vi "Camera.v8.vi"() -> ()   [LabVIEW 2015]
uses:
  Camera Properties.ctl
  Microscope Settings.ctl
  CameraState.ctl
  ModeEnum.ctl
  Stack_State.ctl
  Stack Track.ctl
  CameraControlTypeDef.ctl
  <vilib>/DAQmx/write.llb/DAQmx Write (Digital 1D Wfm NChan NSamp).vi
  <vilib>/DAQmx/write.llb/DAQmx Write (Analog 1D Wfm NChan NSamp).vi
  <vilib>/DAQmx/create/channels.llb/DAQmx Create Channel (DO-Digital Output).vi
  <vilib>/DAQmx/create/channels.llb/DAQmx Create Channel (AO-Voltage-Basic).vi
  <vilib>/Waveform/WDTOps.llb/WDT Number of Waveform Samples DBL.vi
  <vilib>/DAQmx/configure/timing.llb/DAQmx Timing (Sample Clock).vi
  <vilib>/Waveform/DWDTOps.llb/DWDT Uncompress Digital.vi
  <vilib>/DAQmx/miscellaneous.llb/DAQmx Fill In Error Info.vi
  <vilib>/vision/NI_Vision_Development_Module.lvlib
panel:
  in  "Tab Control":enum32{"Camera Settings", "Recording"}(tab)
  in  "?":bool
  in  "Microscope Settings":T1={"Mode"=enum."XY", "Colour 2"={"Laser"=enum."445", "Filter"=0}, "Slit"={"Scanning Mode"=12.0, "Slit Width /%"=5.0}, "Piezo Position /um"=0.0, "Z Axis Stepping"={"Start"=0.0, "Step"=1.0, "End"=100.0}, "Exposure/ms"=40.0, "ROI"={"Height"=2048.0, "Width"=2048.0, "x"=0.0, "y"=0.0}, "Samples per millisecond"=100.0, "Relax/ms"=10.0, "Readout Direction"=2.0, "Trigger Source"=2.0, "Camera Delay"=11.0} {"Colour 2"."Filter" items=["Empty"=1, ""=2, ""=3, "561"=4, ""=5, "488"=6]; "Z Axis Stepping"."End" min=0.0 max=10.0 step=0.05; "Z Axis Stepping"."Step" min=0.0 max=10.0 step=0.05; "Z Axis Stepping"."Start" min=0.0 max=10.0 step=0.05; "ROI"."y" min=0.0 max=10.0 step=0.05; "ROI"."x" min=0.0 max=10.0 step=0.05; "ROI"."Width" min=0.0 max=10.0 step=0.05; "ROI"."Height" min=0.0 max=10.0 step=0.05; "Camera Delay" min=0.0 max=10.0 step=0.05; "Trigger Source" items=["Internal"=1.0, "External"=2.0]; "Readout Direction" items=["Internal"=1.0, "External"=2.0]; "Slit"."Scanning Mode" items=["Full Frame"=1.0, "Slit Scanning"=12.0]; "Piezo Position /um" min=0.0 max=10.0 step=0.05; "Relax/ms" min=0.0 max=10.0 step=0.05}
  in  "Scan":bool
  in  "Scan Continuously":bool
  out "error IO":errorcluster
  in  "Advanced DCAM Controls":i32(listbox) caption="Multicolumn Listbox"
  in  "Properties":T2=4211904 items=["SENSOR MODE"=4212128, "CCD MODE"=4212384, "READOUT MODE"=4211872, "ACTIVE VIEW INDEX"=4343136, "BITS PER CHANNEL"=4342976, "IMAGE PIXEL TYPE"=4343296, "BINNING"=4215968, "EXPOSURE TIME"=2049184, "CONTRAST GAIN"=3163312, "CONTRAST OFFSET"=3163328, "LIGHT MODE"=2114720, "SENSITIVITY"=2114992, "PHOTON IMAGING MODE"=2115200, "HIGH DYNAMIC RANGE MODE"=3163360, "WHITE BALANCE"=3163568, "TEMPERATURE"=2115232, "TEMPERATURE TARGET"=2115264, "SENSOR COOLER FAN"=2115296, "LINEBUNDLE HEIGHT"=4212192, "MECHANICAL SHUTTER"=2115488, "BACK FOCUS POSITION"=8422304, "TRIGGER CONNECTOR"=1066432, "TRIGGER SOURCE"=1066144, "OUTPUT TRIGGER SOURCE"=1852576, "TRIGGER GLOBAL EXPOSURE"=2049680, "FIRST TRIGGER BEHAVIOR"=2049696, "CHANNEL SYNC"=1852352, "READOUT DIRECTION"=4211904, "PRE HSYNC COUNT"=1852704, "INTERNAL LINE SPEED"=4191408, "INTERNAL LINE INVERVAL"=4191424]
  in  "Array":T1[](array[typedef]) {"Colour 2"."Filter" items=["Empty"=1, ""=2, ""=3, "561"=4, ""=5, "488"=6]; "Z Axis Stepping"."End" min=0.0 max=10.0 step=0.05; "Z Axis Stepping"."Step" min=0.0 max=10.0 step=0.05; "Z Axis Stepping"."Start" min=0.0 max=10.0 step=0.05; "ROI"."y" min=0.0 max=10.0 step=0.05; "ROI"."x" min=0.0 max=10.0 step=0.05; "ROI"."Width" min=0.0 max=10.0 step=0.05; "ROI"."Height" min=0.0 max=10.0 step=0.05; "Camera Delay" min=0.0 max=10.0 step=0.05; "Trigger Source" items=["Internal"=1.0, "External"=2.0]; "Readout Direction" items=["Internal"=1.0, "External"=2.0]; "Slit"."Scanning Mode" items=["Full Frame"=1.0, "Slit Scanning"=12.0]; "Piezo Position /um" min=0.0 max=10.0 step=0.05; "Relax/ms" min=0.0 max=10.0 step=0.05}
  out "Image":T3(plugin-control)
  out "Histogram":T4(graph)
  in  "stop":bool
  in  "Signals Debugger":bool
  in  "Calibration":bool
  in  "MultiD Scan":bool
  in  "Stage Controller":bool
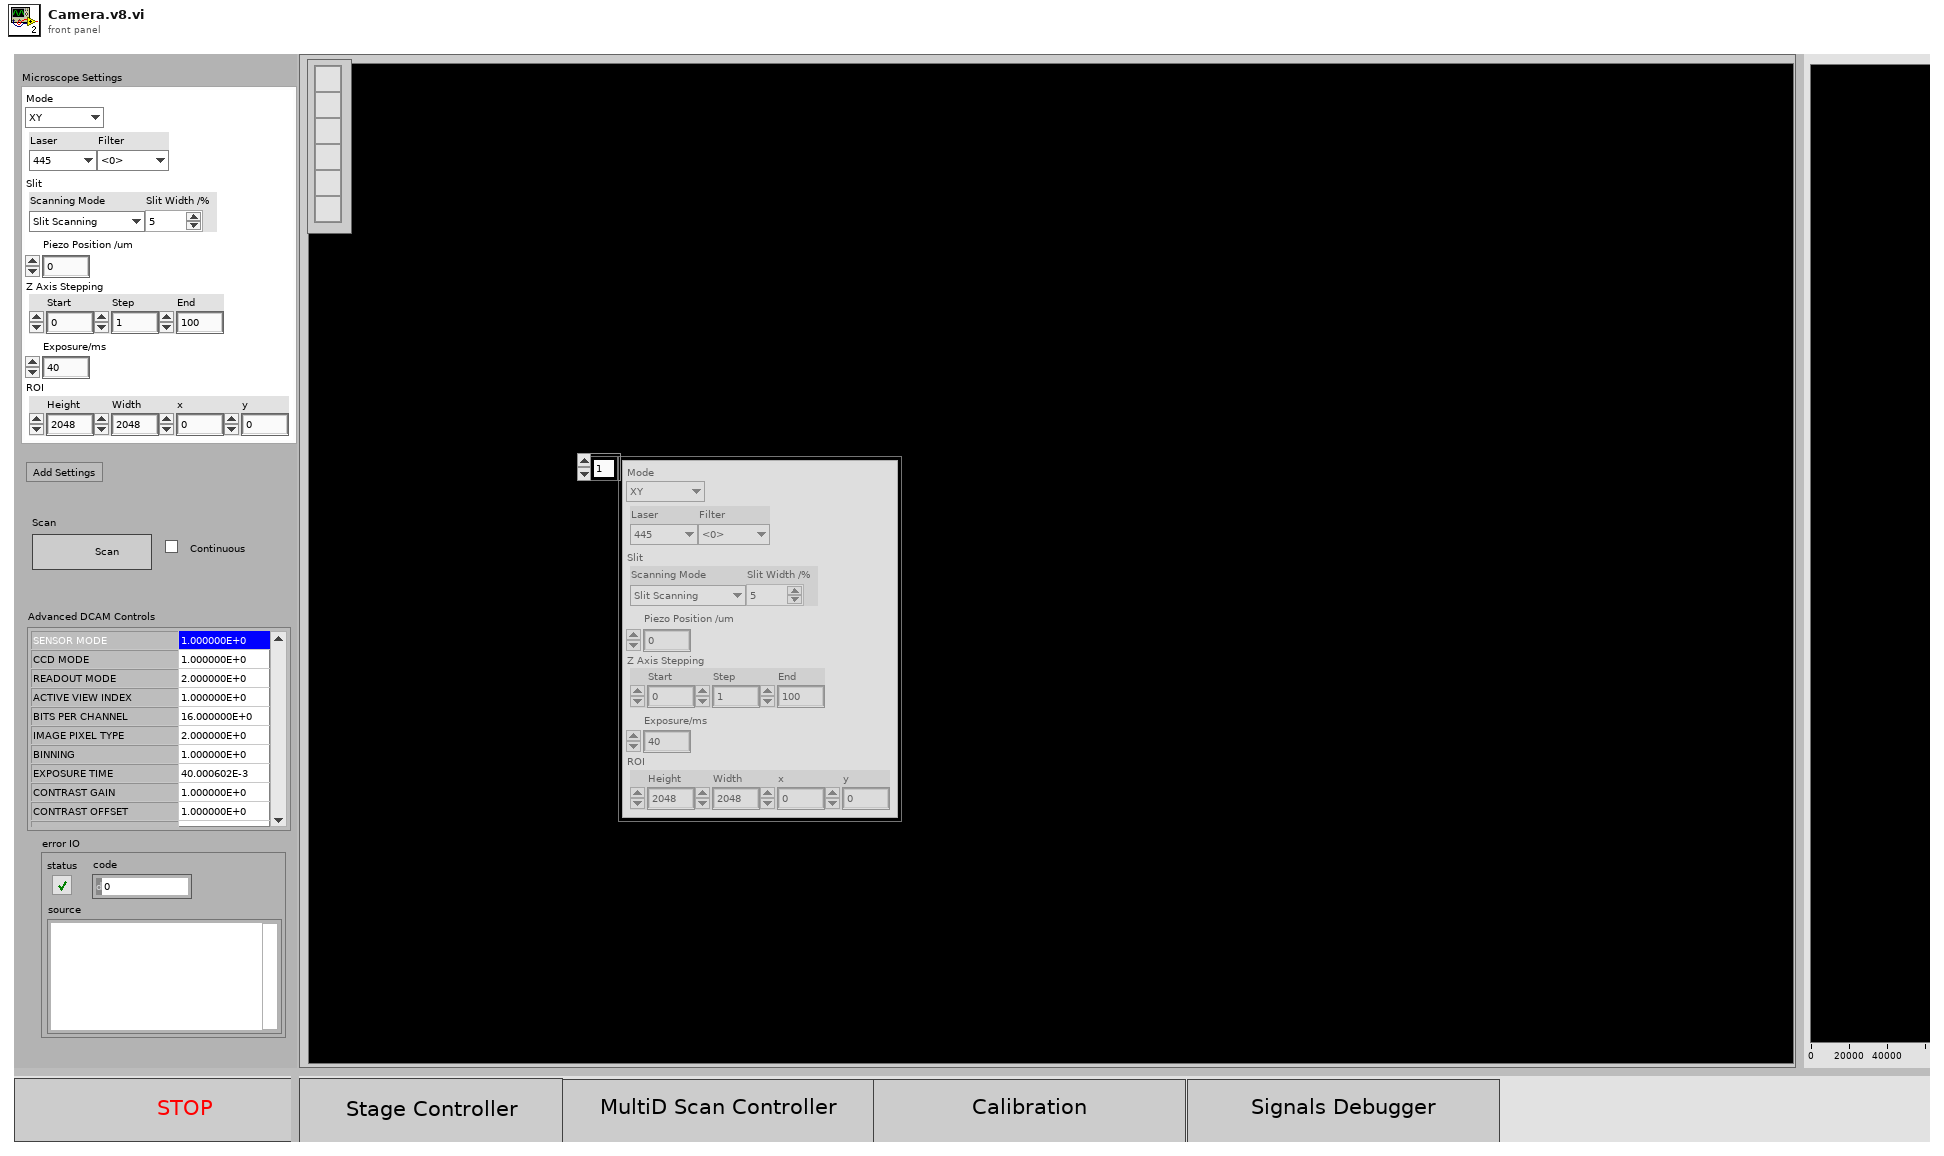
[diagram p1: front panel]
types:
  T1 = typedef "Microscope Settings.ctl" = cluster{"Mode":enum16{"X", "XY", "XYZ", "XYZT", "XYZC"}, "Colour 2":cluster{"Laser":enum16{"445", "488", "561", "647"}, "Filter":u16}, "Slit":cluster{"Scanning Mode":dbl, "Slit Width /%":dbl}, "Piezo Position /um":dbl, "Z Axis Stepping":cluster{"Start":dbl, "Step":dbl, "End":dbl}, "Exposure/ms":dbl, "ROI":cluster{"Height":dbl, "Width":dbl, "x":dbl, "y":dbl}, "Samples per millisecond":dbl, "Relax/ms":dbl, "Readout Direction":dbl, "Trigger Source":dbl, "Camera Delay":dbl}
  T2 = typedef "Camera Properties.ctl" = u32
  T3 = typedef "IMAQ Image.ctl" = refnum<image>
  T4 = cluster{"Starting Value":sgl, "Incremental Value":sgl, "Histogram":u32[]}
  T5 = cluster{"height":u32, "width":u32, "datatype":u32}
  T6 = typedef "CameraState.ctl" = enum16{"init", "active", "deinit"}
  T7 = typedef "ModeEnum.ctl" = enum16{"Idle", "generateWaves", "runWaves", "stop"}
  T8 = typedef "CameraControlTypeDef.ctl" = enum16{"Idle", "IntervalLineInt", "Ram Record", "HardDisk Record", "Disengage Update", "Update", "ROI", "Binning", "Scan Mode", "Trigger Mode", "Readout Mode", "Readout Direction", "Preview", "ROIWindow", "Trigger Source"}
  T9 = cluster{"Mode":u32, "Polarity":u32, "Times":u32, "Delay":dbl}
  T10 = typedef "Stack_State.ctl" = cluster{"State":T11, "Stack Number":i32, "Image":u16[][], "Stacks":i32}
  T11 = typedef "Stack Track.ctl" = enum16{"Idle", "Display", "Start Sequence", "Read Disk", "STOP", "Collecting", "End"}
  T12 = enum32{"Invalid", "Standard", "Closed", "Hidden", "Minimized", "Maximized"}
  T13 = typedef "Image Type" = u32
  T14 = cluster{"State":T11, "Timeout":i32, "Data 16":u16[][], "Timeout":i32}
  T15 = cluster{waveform(dbl)[], "Digital Waveform":digitalwaveform, "Digital Waveform":digitalwaveform}
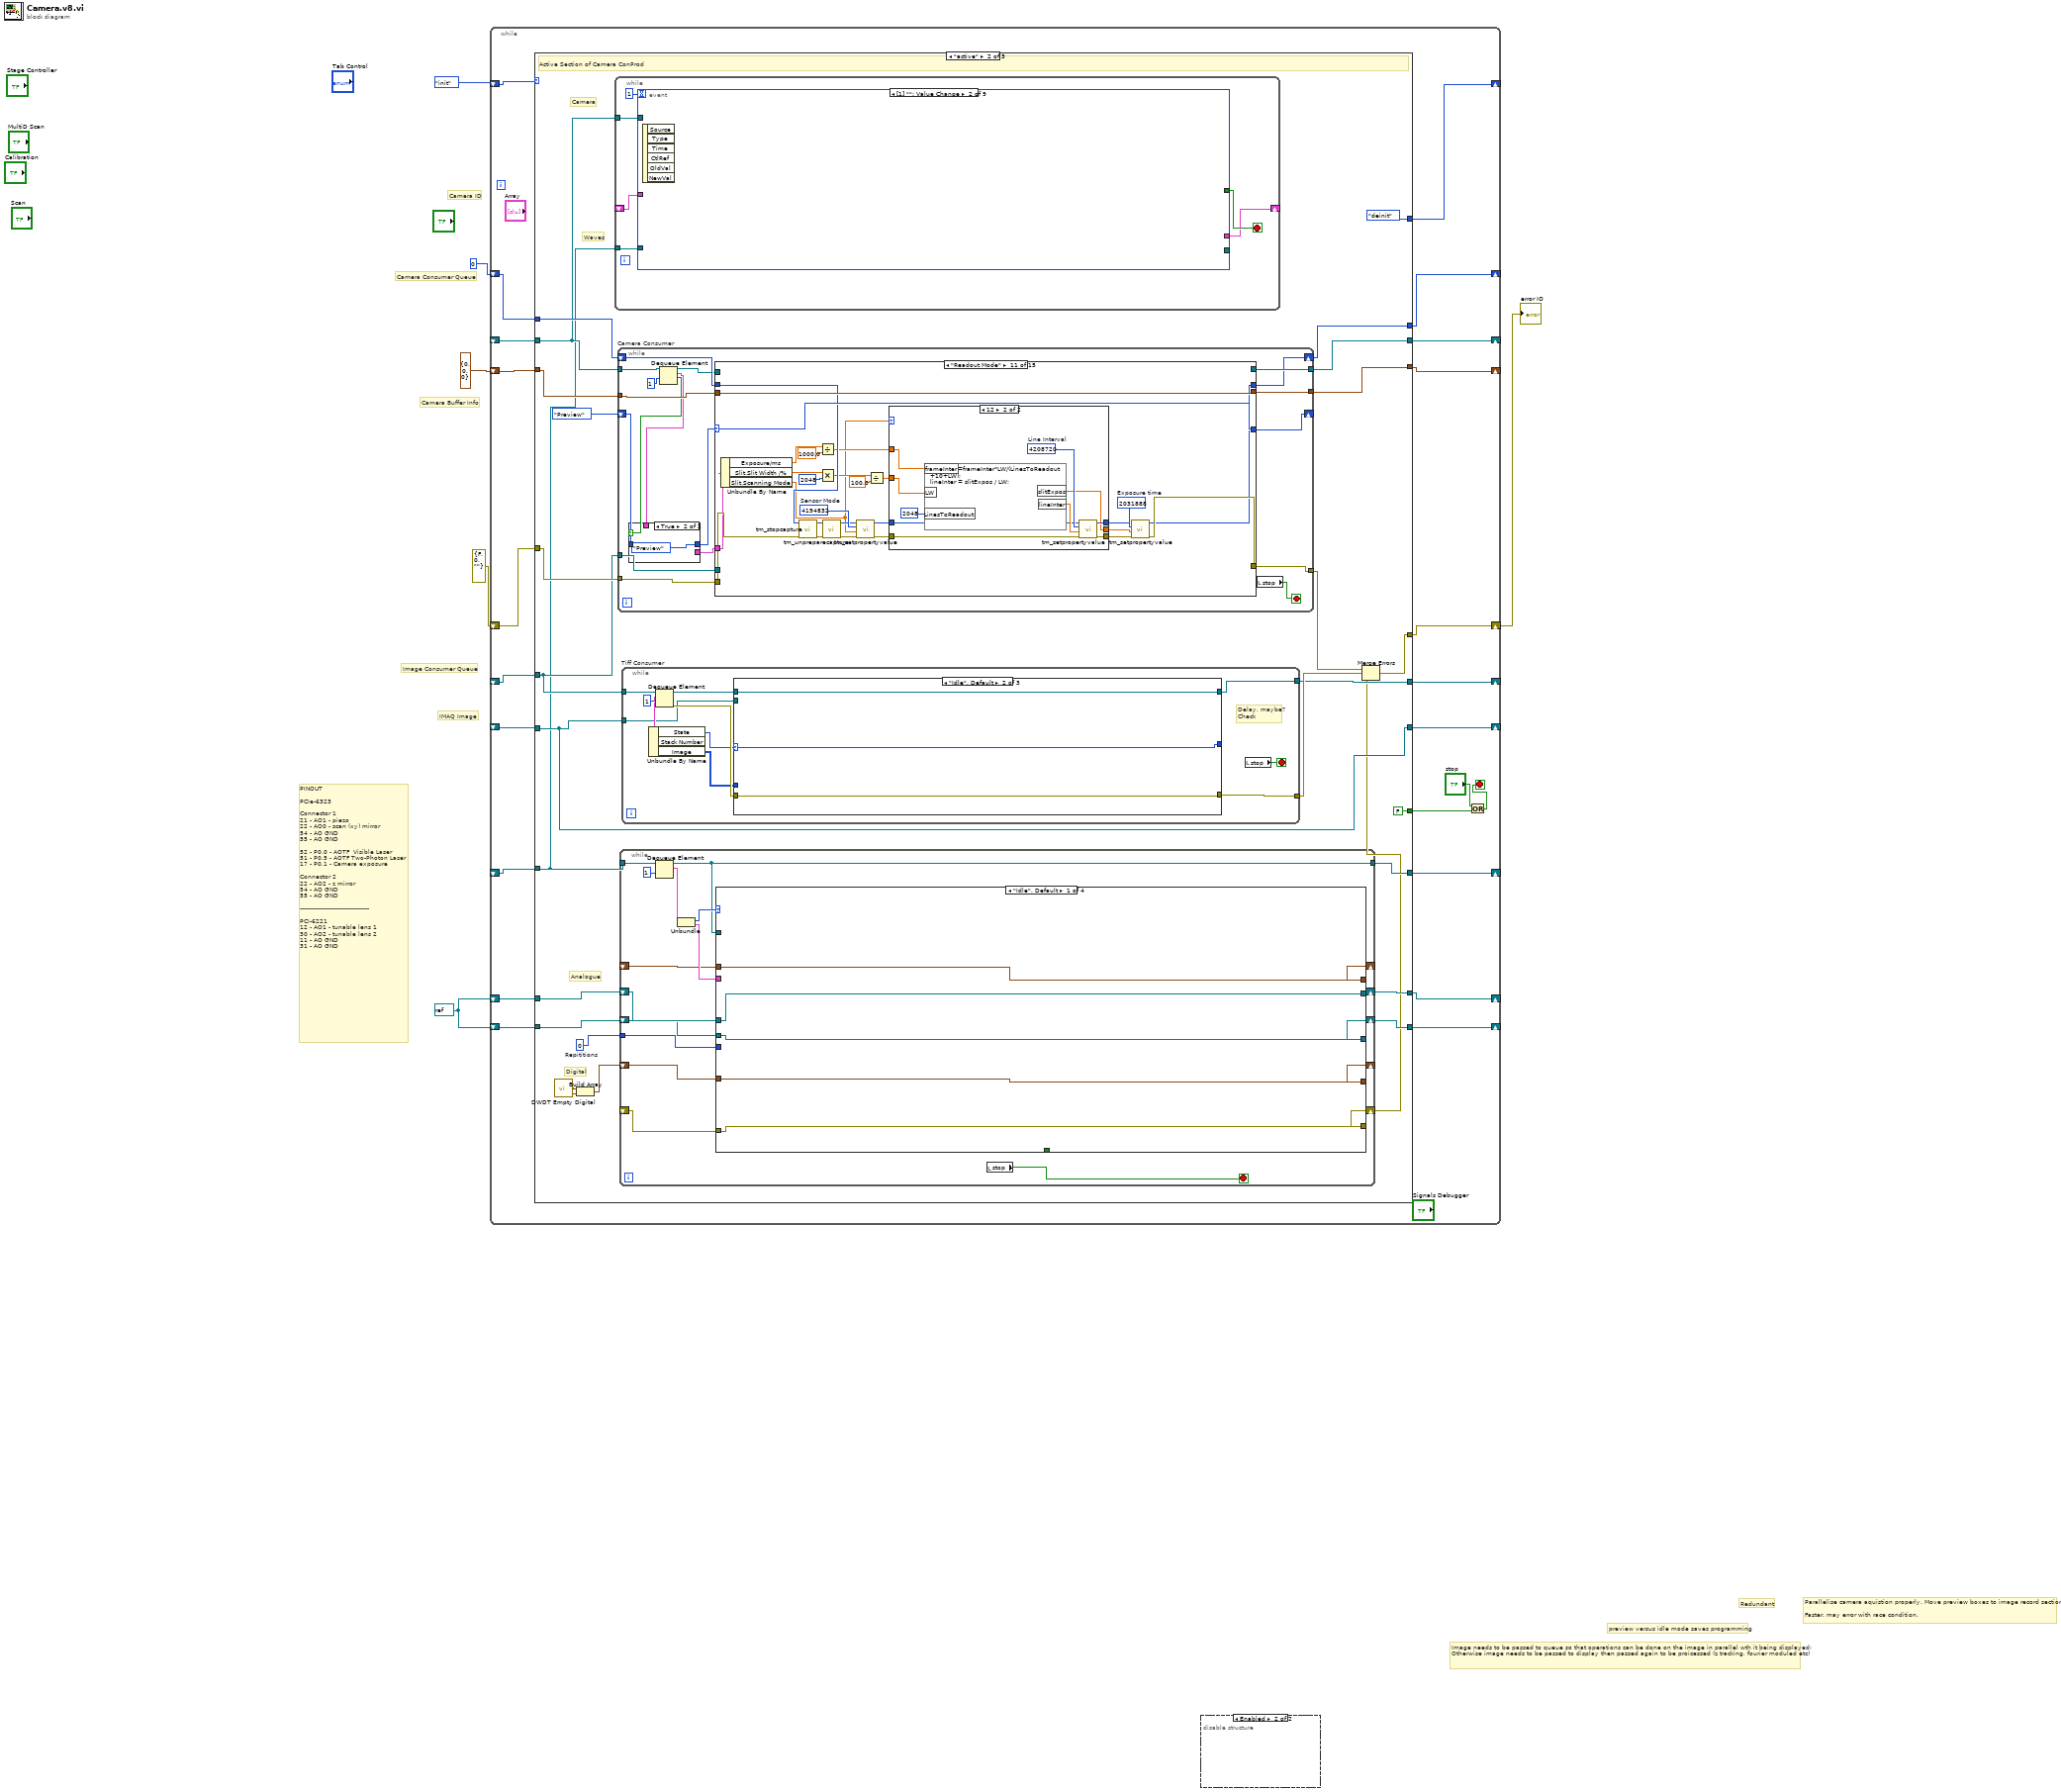
[diagram p0: block diagram]
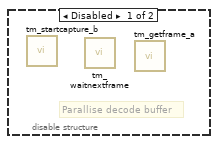
[diagram p2: hidden frame]
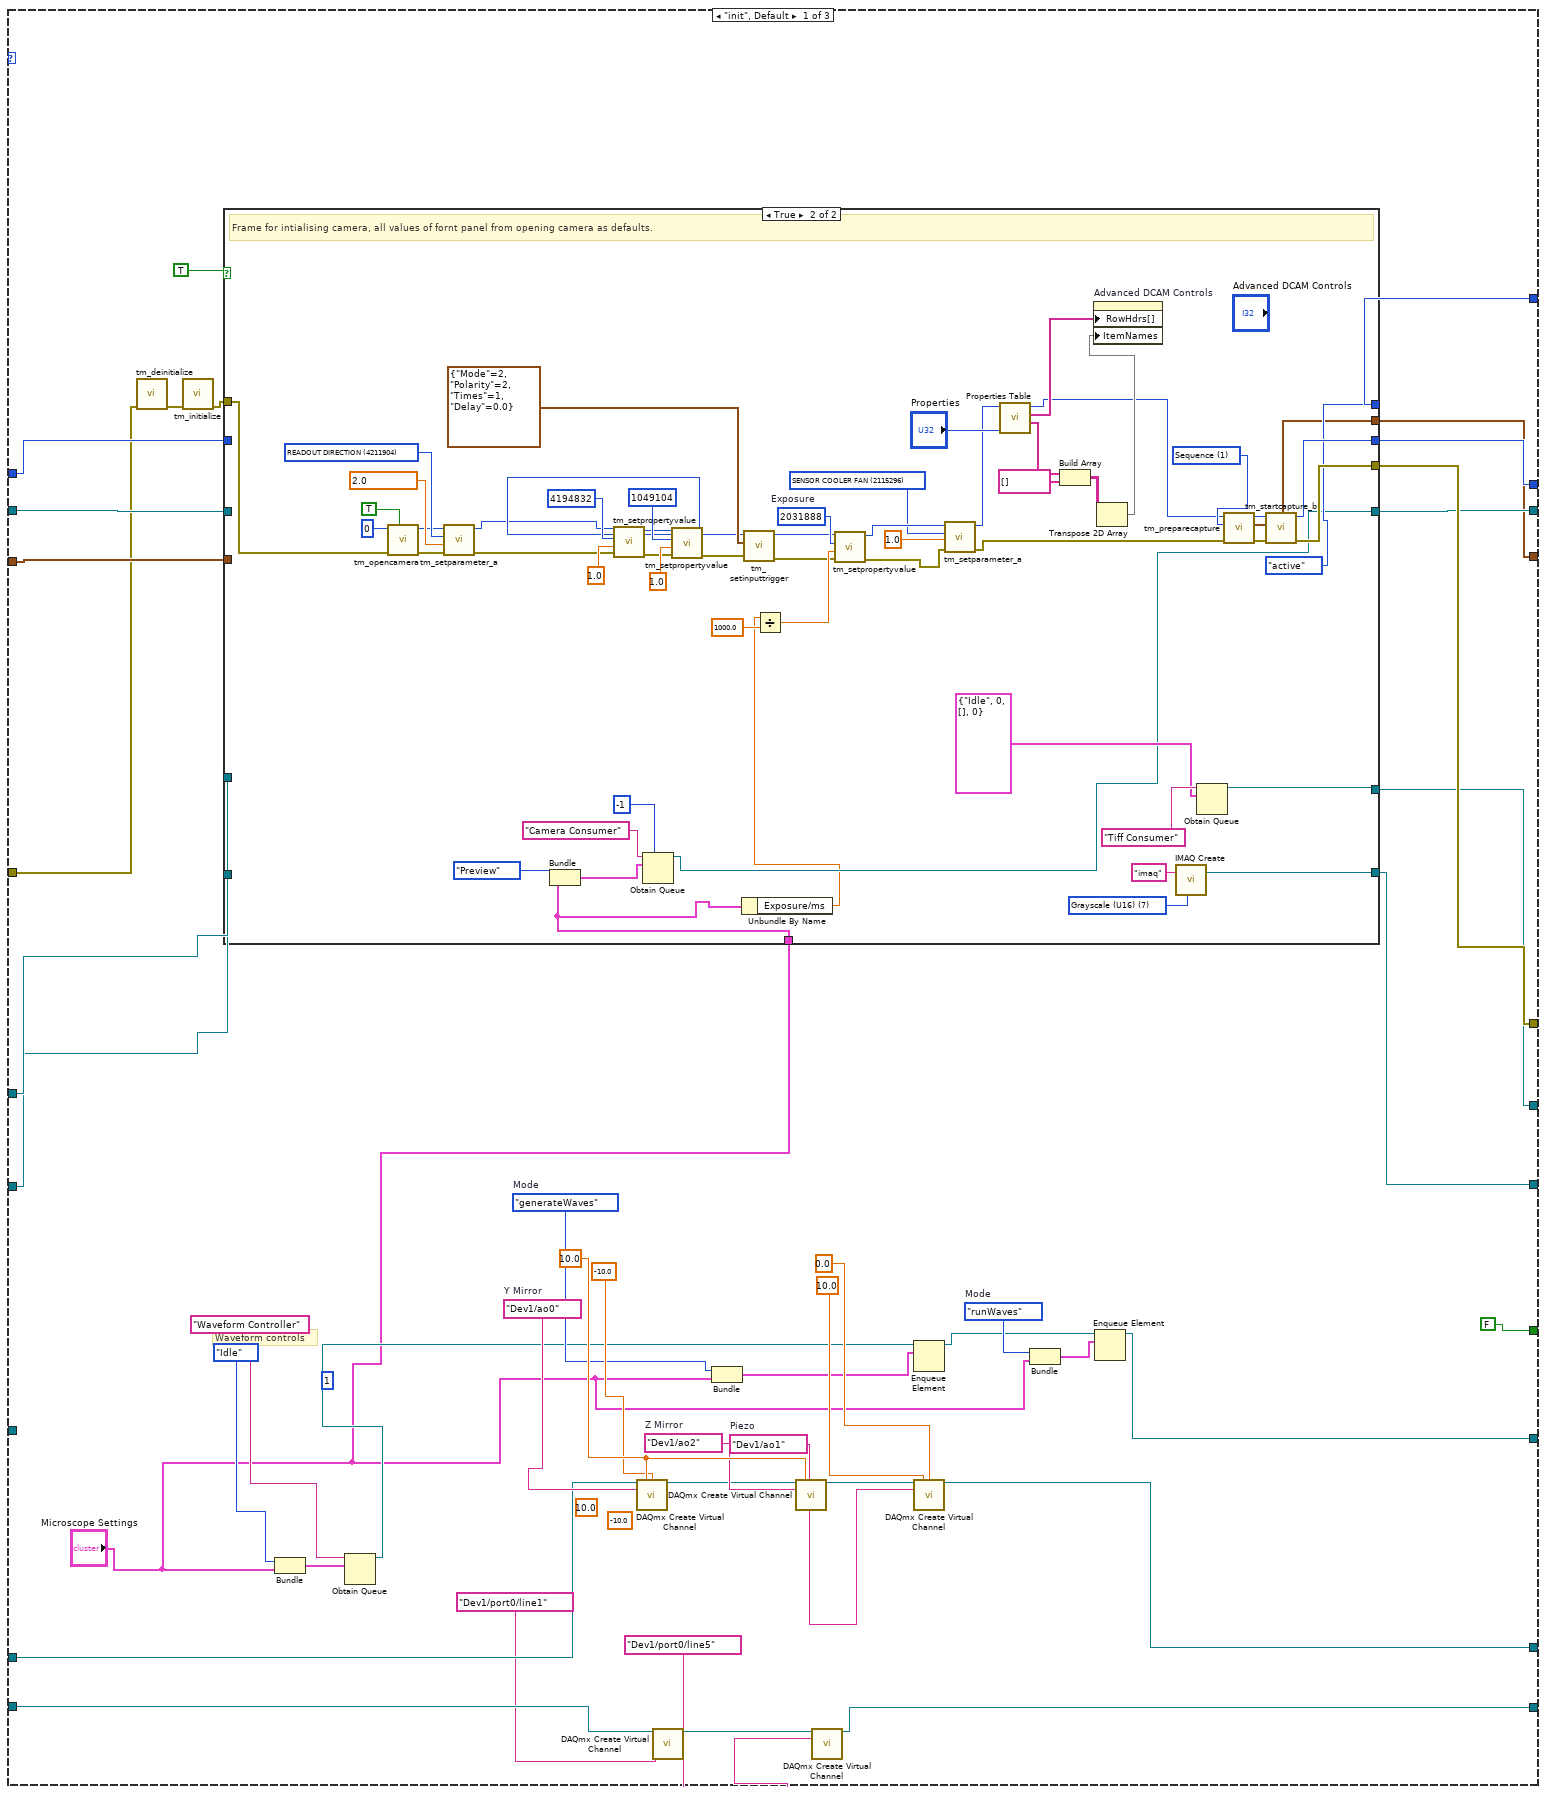
[diagram p3: hidden frame]
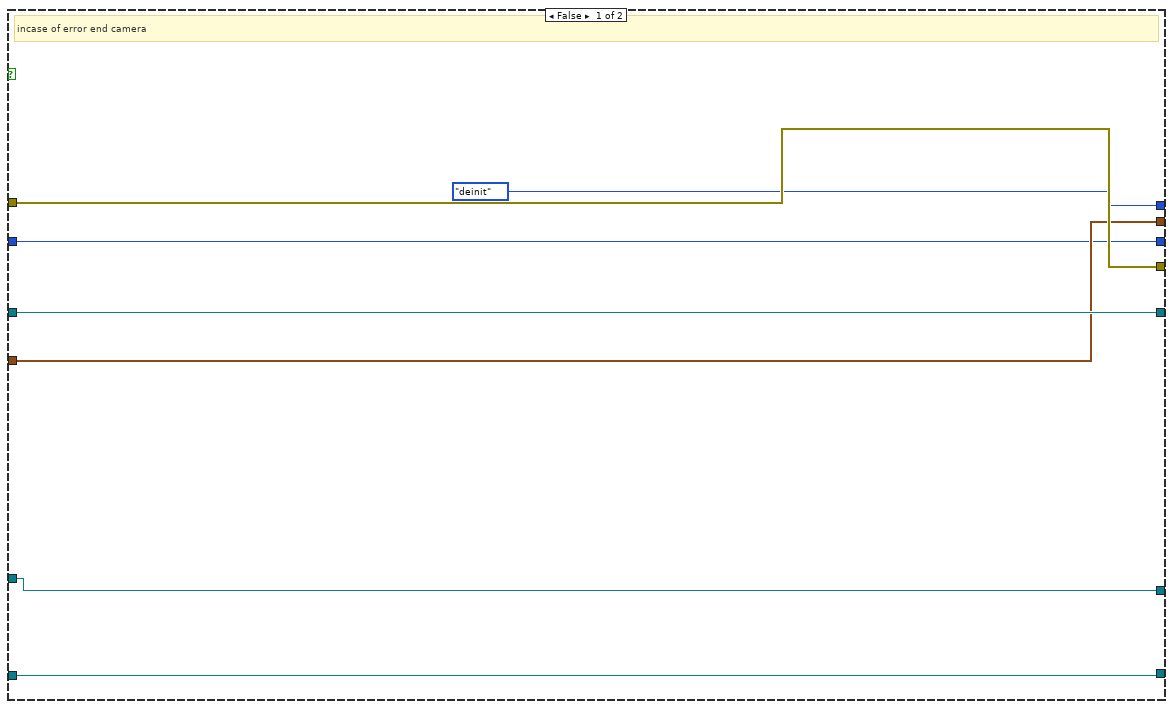
[diagram p4: hidden frame]
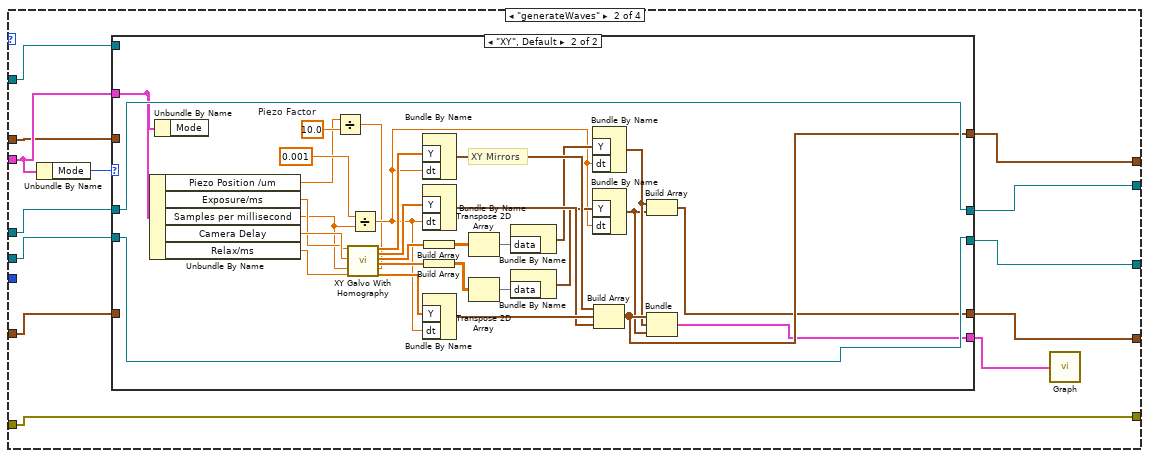
[diagram p5: hidden frame]
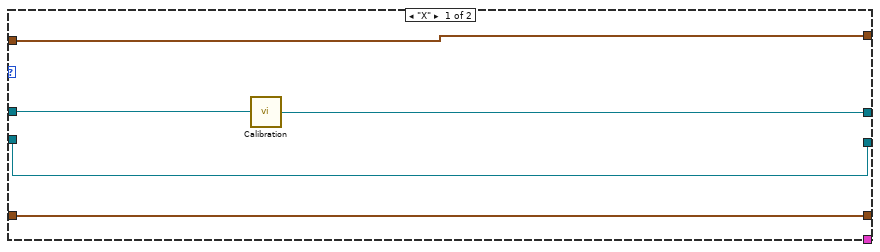
[diagram p6: hidden frame]
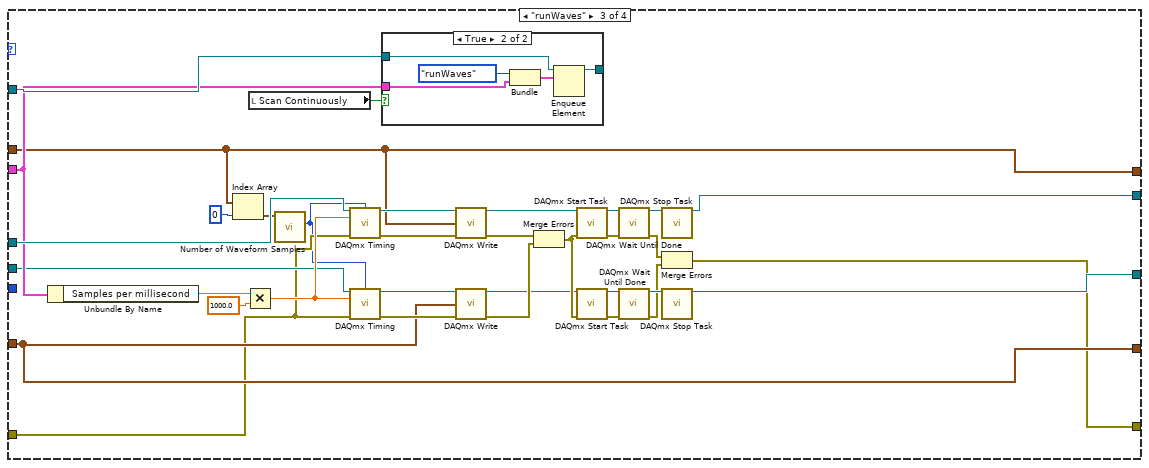
[diagram p7: hidden frame]
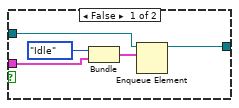
[diagram p8: hidden frame]
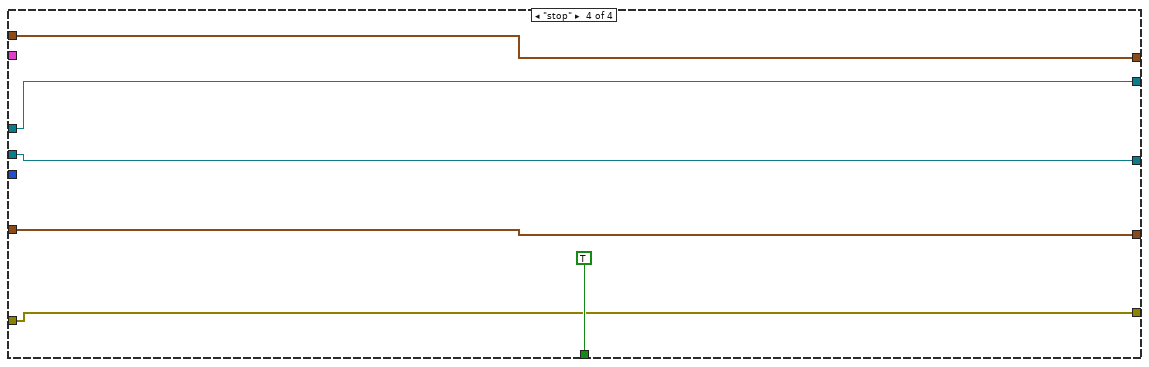
[diagram p9: hidden frame]
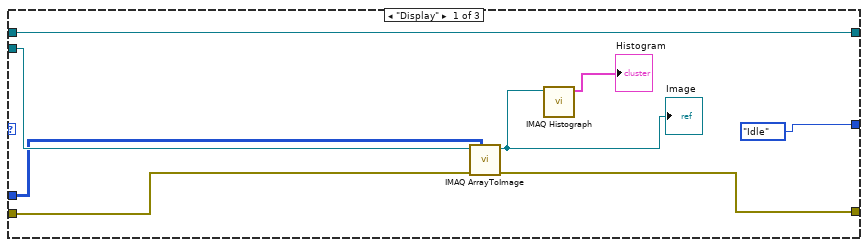
[diagram p10: hidden frame]
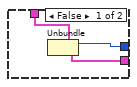
[diagram p12: hidden frame]
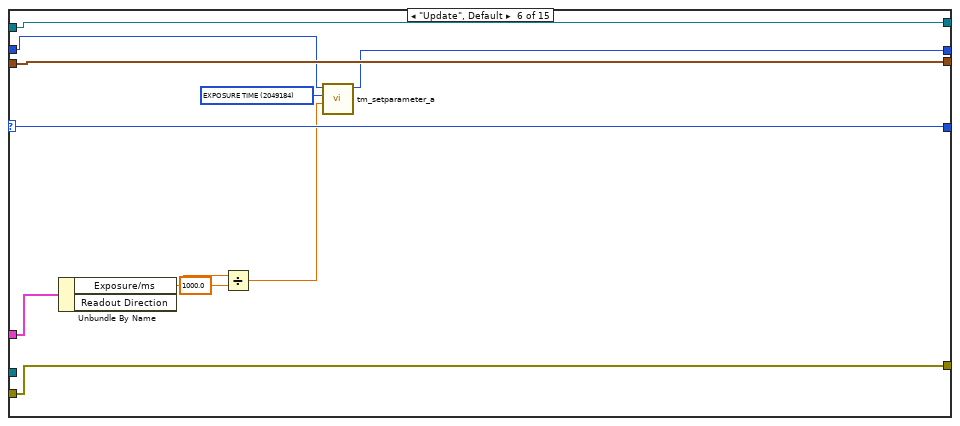
[diagram p18: hidden frame]
diagram:
  w3 = refnum<k21> refnum ("Mirror Z 2")
  # "PINOUT\n\nPCIe-6323\n\nConnector 1\n21 - AO1 - piezo\n22 - AO0 - scan (xy) mirror\n54 - AO GND\n55 - AO GND\n\n52 - P0.0 - AOTF  Visible Laser\n51 - P0.5 - AOTF Two-Photon Laser\n17 - P0.1 - Camera exposure\n\nConnector 2\n22 - AO2 - z mirror\n54 - AO GND\n55 - AO GND\n\n-----------------------------------\n\nPCI-6221\n12 - AO1 - tunable lens 1\n30 - AO2 - tunable lens 2\n11 - AO GND\n31 - AO GND"
  # "IMAQ Image"
  # "Camera Buffer Info"
  # "Image needs to be passed to queue so that operations can be done on the image in parallel wth it being displayed;\nOtherwise image needs to be passed to display then passed again to be proicessed (z tracking, fourier moduled etc)"
  # "preview versus idle mode saves programming"
  # "Parallelise camera aquistion properly. Move preview boxes to image record section.\n\nFaster. may error with race condition."
  # "Redundant"
  # "Image Consumer Queue"
  # "Camera Consumer Queue"
  # "Camera ID"
  n1 = while {
    shift-right: [w29] -> _
    shift-left: CameraState."init" -> [w28]
    shift-right: [w27] -> _
    shift-left: u32 0 ("Handle out") -> [w26]
    shift-right: [w25] -> w5
    shift-left: errorcluster {"status"=FALSE, "code"=0, "source"=""} ("error IO") -> [w24]
    shift-right: [w22] -> _
    shift-left: _ -> [w21]
    shift-right: [w23] -> _
    shift-left: _ -> [w20]
    shift-right: [w16] -> _
    shift-left: T5 {"height"=0, "width"=0, "datatype"=0} ("Buffer Info") -> [w15]
    shift-right: [w14] -> _
    shift-left: _ -> [w13]
    shift-right: [w12] -> _
    shift-left: w3 -> [w11]
    shift-right: [w9] -> _
    shift-left: w3 -> [w10]
    shift-right: [w8] -> _
    shift-left: _ -> [w7]
    stop <- w18 stop-if-true
    n2 = case shown="\"active\"" w28 {
      tunnel: [w71 CameraState."deinit" CameraState."init"] -> w29
      tunnel: [w70 w161 w563] -> w27
      tunnel: w26 -> [w48 w162 w563]
      tunnel: [w69 w160 w566] -> w25
      tunnel: w24 -> [w47 w154 w567]
      tunnel: [w68 w157 w550] -> w23
      tunnel: [w67 w156 w546] -> w22
      tunnel: w21 -> [w65 w149 w546]
      tunnel: w20 -> [w66 w147 w550]
      tunnel: [FALSE ("stop") FALSE ("stop") TRUE ("stop")] -> w17
      tunnel: [w63 w152 w560] -> w16
      tunnel: w15 -> [w62 w151 w560]
      tunnel: w13 -> [w60 w148 w559]
      tunnel: [w61 w148 w559] -> w14
      tunnel: w7 -> [_ w139 w545]
      tunnel: [w52 w140 w557] -> w12
      tunnel: w11 -> [w49 w143 w557]
      tunnel: w10 -> [w45 w142 w555]
      tunnel: [w40 w141 w555] -> w9
      tunnel: [w30 w138 w545] -> w8
      frame "init", Default {
        w35 = ModeEnum."runWaves"  # Mode
        (unwired) 1 ("max queue size (-1, unlimited)")
        w44 = ModeEnum."generateWaves"  # Mode
        (unwired) -10.0 ("minimum value")
        (unwired) 10.0 ("maximum value")
        w55 = tag "Dev1/ao1"  # Piezo
        w56 = tag "Dev1/ao2"  # Z Mirror
        w57 = tag "Dev1/ao0"  # Y Mirror
        w59 = 10.0 ("maximum value")
        # "Waveform controls"
        n3 = call "tm_deinitialize.vi"("error in (no error)"=w47) -> ("error out"=w73:errorcluster)  [unwired: 10 in]
        n4 = call "tm_initialize.vi"("error in (no error)"=w73) -> ("error out"=w72:errorcluster)  [unwired: 7 in, 3 out]
        n5 = case shown="True" TRUE {
          tunnel: w72 -> [w80 w101]
          tunnel: [CameraState."deinit" CameraState."active"] -> w71
          tunnel: [w80 w132] -> w69
          tunnel: [w75 w130] -> w70
          tunnel: [w78 w120] -> w68
          tunnel: [w77 w127] -> w67
          tunnel: w66 -> [w78 _]
          tunnel: w65 -> [w77 _]
          tunnel: [w76 w125] -> w63
          tunnel: w62 -> [w76 _]
          tunnel: w48 -> [w75 _]
          tunnel: [w74 w122] -> w61
          tunnel: w60 -> [w74 _]
          tunnel: "Microscope Settings" -> [_ w88]
          frame False {
            # "incase of error end camera"
          }
          frame True {
            w98 = u32 2115296 items=["SENSOR MODE"=4212128, "CCD MODE"=4212384, "READOUT MODE"=4211872, "ACTIVE VIEW INDEX"=4343136, "BITS PER CHANNEL"=4342976, "IMAGE PIXEL TYPE"=4343296, "BINNING"=4215968, "EXPOSURE TIME"=2049184, "CONTRAST GAIN"=3163312, "CONTRAST OFFSET"=3163328, "LIGHT MODE"=2114720, "SENSITIVITY"=2114992, "PHOTON IMAGING MODE"=2115200, "HIGH DYNAMIC RANGE MODE"=3163360, "WHITE BALANCE"=3163568, "TEMPERATURE"=2115232, "TEMPERATURE TARGET"=2115264, "SENSOR COOLER FAN"=2115296, "LINEBUNDLE HEIGHT"=4212192, "MECHANICAL SHUTTER"=2115488, "BACK FOCUS POSITION"=8422304, "TRIGGER CONNECTOR"=1066432, "TRIGGER SOURCE"=1066144, "OUTPUT TRIGGER SOURCE"=1852576, "TRIGGER GLOBAL EXPOSURE"=2049680, "FIRST TRIGGER BEHAVIOR"=2049696, "CHANNEL SYNC"=1852352, "READOUT DIRECTION"=4211904, "PRE HSYNC COUNT"=1852704, "INTERNAL LINE SPEED"=4226000, "INTERNAL LINE INTERVAL"=4226016] ("Parameter")
            w107 = u32 2031888  # Exposure
            w118 = sgl 2.0 items=["Forward"=1.0, "Backward"=2.0] ("Readout Direction")
            w119 = u32 4211904 items=["SENSOR MODE"=4212128, "CCD MODE"=4212384, "READOUT MODE"=4211872, "ACTIVE VIEW INDEX"=4343136, "BITS PER CHANNEL"=4342976, "IMAGE PIXEL TYPE"=4343296, "BINNING"=4215968, "EXPOSURE TIME"=2049184, "CONTRAST GAIN"=3163312, "CONTRAST OFFSET"=3163328, "LIGHT MODE"=2114720, "SENSITIVITY"=2114992, "PHOTON IMAGING MODE"=2115200, "HIGH DYNAMIC RANGE MODE"=3163360, "WHITE BALANCE"=3163568, "TEMPERATURE"=2115232, "TEMPERATURE TARGET"=2115264, "SENSOR COOLER FAN"=2115296, "LINEBUNDLE HEIGHT"=4212192, "MECHANICAL SHUTTER"=2115488, "BACK FOCUS POSITION"=8422304, "TRIGGER CONNECTOR"=1066432, "TRIGGER SOURCE"=1066144, "OUTPUT TRIGGER SOURCE"=1852576, "TRIGGER GLOBAL EXPOSURE"=2049680, "FIRST TRIGGER BEHAVIOR"=2049696, "CHANNEL SYNC"=1852352, "READOUT DIRECTION"=4211904, "PRE HSYNC COUNT"=1852704, "INTERNAL LINE SPEED"=4226000, "INTERNAL LINE INTERVAL"=4226016] ("Parameter")
            w124 = T13 7 items=["Grayscale (U8)", "Grayscale (I16)", "Grayscale (SGL)", "Complex (CSG)", "RGB (U32)", "HSL (U32)", "RGB (U64)", "Grayscale (U16)"] ("Image Type")
            w134 = 1 items=["Snap", "Sequence"] ("Capture mode")
            # "Frame for intialising camera, all values of fornt panel from opening camera as defaults."
            n6 = call "tm_opencamera.vi"("Force Open"=TRUE, "error in (no error)"=w101, "Camera Index"=u32 0) -> ("error out"=w116:errorcluster, "Handle out"=w117:u32)  [unwired: 6 in, 1 out]
            n7 = call "tm_setparameter_a.vi"("error in (no error)"=w116, "Value in"=w118, "Parameter"=w119, "Handle in"=w117) -> ("error out"=w86:errorcluster, "Handle out"=w108:u32)  [unwired: 6 in]
            n8 = Bundle("Enum"=CameraControlTypeDef."Preview", "Microscope Settings"=w88) -> (w102:cluster{"Enum":T8, "Microscope Settings":T1})  [unwired: 1 in]
            n9 = call "tm_setpropertyvalue.vi"("error in (no error)"=w86, "Value in"=sgl 1.0, "Property ID"=u32 4194832, "Handle in"=w108) -> ("error out"=w85:errorcluster, "Handle out"=w111:u32)  [unwired: 6 in]
            n10 = Obtain Queue(max queue size (-1, unlimited)=-1, name (unnamed)="Camera Consumer", element data type=w102) -> (queue out=w120:refnum<queue>)  [unwired: 2 in, 2 out]
            n11 = call "tm_setpropertyvalue.vi"("error in (no error)"=w85, "Value in"=sgl 1.0, "Property ID"=u32 1049104, "Handle in"=w111) -> ("error out"=w84:errorcluster, "Handle out"=w109:u32)  [unwired: 6 in]
            n12 = Unbundle By Name(w88) -> ("Exposure/ms"=w87:dbl)
            n13 = call <userlib>:"tm_setinputtrigger.vi"("error in (no error)"=w84, "Parameters"=T9 {"Mode"=2, "Polarity"=2, "Times"=1, "Delay"=0.0}, "Handle in"=w109) -> ("error out"=w83:errorcluster, "Handle out"=w106:u32)  [unwired: 7 in]
            n14 = Divide(x=w87, y=sgl 1000.0) -> (x/y=w104:dbl)
            n15 = call "tm_setpropertyvalue.vi"("error in (no error)"=w83, "Value in"=w104, "Property ID"=w107, "Handle in"=w106) -> ("error out"=w82:errorcluster, "Handle out"=w99:u32)  [unwired: 6 in]
            n16 = call "tm_setparameter_a.vi"("error in (no error)"=w82, "Value in"=1.0, "Parameter"=w98, "Handle in"=w99) -> ("error out"=w81:errorcluster, "Handle out"=w90:u32)  [unwired: 6 in]
            n17 = call "Properties Table.vi"("Properties"="Properties", "Handle In"=w90) -> ("Value Stirngs Out"=w94:string[], "Row Headers"=w95:string[], "Handle Out"=w89:u32)  [unwired: 3 in, 1 out]
            n18 = Build Array(w94, string[] [] ("element")) -> (w92:string[][])
            n19 = Transpose 2D Array(2D array=w92) -> (transposed array=w91:string[][])
            n20 = property on="Advanced DCAM Controls" class="MCListbox (strict)"("RowHdrs[]"=w95, "ItemNames"=w91) -> ()  [unwired: 2 in, 2 out]
            n21 = call "IMAQ Create"("Image Name"="imaq", "Image Type"=w124) -> ("New Image"=w122:T3)  [unwired: 3 in, 1 out]
            n22 = Obtain Queue(name (unnamed)="Tiff Consumer", element data type=T10 {"State"=enum."Idle", "Stack Number"=0, "Image"=[], "Stacks"=0} ("input cluster")) -> (queue out=w127:refnum<queue>)  [unwired: 3 in, 2 out]
            n23 = call "tm_preparecapture.vi"("error in (no error)"=w81, "Capture mode"=w134, "Handle in"=w89) -> ("error out"=w133:errorcluster, "Buffer Info"=w125:T5, "Handle out"=w131:u32)  [unwired: 5 in, 1 out]
            n24 = call "tm_startcapture_b.vi"("error in (no error)"=w133, "Handle in"=w131) -> ("error out"=w132:errorcluster, "Handle out"=w130:u32)  [unwired: 8 in]
          }
        }
        n25 = Bundle("Mode"=ModeEnum."Idle", "Microscope Settings"="Microscope Settings") -> (w42:cluster{"Mode":T7, "Microscope Settings":T1})  [unwired: 1 in]
        n26 = Obtain Queue(name (unnamed)="Waveform Controller", element data type=w42) -> (queue out=w41:refnum<queue>)  [unwired: 3 in, 2 out]
        n27 = call-poly <vilib>:"DAQmx Create Virtual Channel.vi"("task in"=w49, "maximum value"=w59, "minimum value"=-10.0, "physical channels"=w57) -> ("task out"=w51:refnum<k21>)  [unwired: 10 in, 1 out]
        n28 = call-poly <vilib>:"DAQmx Create Virtual Channel.vi"("task in"=w45, "lines"=tag "Dev1/port0/line1") -> ("task out"=w46:refnum<k21>)  [unwired: 12 in, 1 out]
        n29 = Bundle("Mode"=w44, "Microscope Settings"="Microscope Settings") -> (w33:cluster{"Mode":T7, "Microscope Settings":T1})  [unwired: 1 in]
        n30 = call-poly <vilib>:"DAQmx Create Virtual Channel.vi"("task in"=w51, "maximum value"=w59, "physical channels"=w56) -> ("task out"=w50:refnum<k21>)  [unwired: 11 in, 1 out]
        n31 = call-poly <vilib>:"DAQmx Create Virtual Channel.vi"("task in"=w46, "lines"=tag "Dev1/port0/line5") -> ("task out"=w40:refnum<k21>)  [unwired: 12 in, 1 out]
        n32 = Enqueue Element(queue=w41, element=w33) -> (queue out=w34:refnum<queue>)  [unwired: 2 in, 2 out]
        n33 = call-poly <vilib>:"DAQmx Create Virtual Channel.vi"("task in"=w50, "maximum value"=10.0 ("minimum value"), "minimum value"=0.0 ("maximum value"), "physical channels"=w55) -> ("task out"=w52:refnum<k21>)  [unwired: 10 in, 1 out]
        n34 = Bundle("Mode"=w35, "Microscope Settings"="Microscope Settings") -> (w31:cluster{"Mode":T7, "Microscope Settings":T1})  [unwired: 1 in]
        n35 = Enqueue Element(queue=w34, element=w31) -> (queue out=w30:refnum<queue>)  [unwired: 2 in, 2 out]
      }
      frame "active" {
        w146 = 0  # Repititions
        # "Waves"
        # "Camera"
        # "Digital"
        # "Analogue"
        # "Active Section of Camera ConProd"
        n36 = call <vilib>:"DWDT Empty Digital.vi"() -> ("digital waveform out"=w144:digitalwaveform)  [unwired: 5 in]
        n37 = Build Array(w144, w144) -> (w145:digitalwaveform[])
        n38 = while {
          tunnel: w147 -> [w497]
          shift-right: [w496] -> _
          shift-left: _ -> [w495]
          tunnel: w139 -> [w493]
          stop <- w498 stop-if-true
          n39 = event shown="[1] \"\": Value Change" {
            selector: _ -> [_ _ _ _ _ _ _ _ _]
            dyn-events: _ -> [_ _ _ _ _ _ _ _ _]
            timeout: 1 -> [_ _ _ _ _ _ _ _ _]
            tunnel: [w506 _ _ _ _ _ _ _ _] -> w498
            tunnel: w497 -> [w501 _ w513 w517 _ w524 _ _ _]
            tunnel: [w499 _ w507 w515 _ _ _ _ w544] -> w496
            tunnel: w495 -> [w499 _ w507 w515 w520 w525 _ w537 _]
            tunnel: [_ _ _ w516 _ _ _ w536 _] -> _
            tunnel: w493 -> [w500 _ w512 w516 w519 w523 _ w535 _]
            event "stop": Value Change {
              w504 = ModeEnum."stop"  # Mode
              n40 = event-data() -> ()  [unwired: 1 in, 6 out]
              n41 = Bundle("Enum"=CameraControlTypeDef."Idle", "Value"=w499) -> (w502:cluster{"Enum":T8, "Value":T1})  [unwired: 1 in]
              n42 = Bundle("Mode"=w504, "Value"=w499) -> (w503:cluster{"Mode":T7, "Value":T1})  [unwired: 1 in]
              n43 = Enqueue Element(queue=w501, element=w502) -> ()  [unwired: 2 in, 3 out]
              n44 = Enqueue Element(queue=w500, element=w503) -> ()  [unwired: 2 in, 3 out]
              n45 = local read "stop"() -> (w506:bool)
            }
            event Value Change {
              n46 = event-data() -> ()  [unwired: 1 in, 6 out]
            }
            event Value Change {
              w510 = ModeEnum."generateWaves"  # Mode
              # "Live video for Calibration and 2D\nScan Modes.\n\nIdle Video for MultiD Scan modes\nUNTIL Begin Scan Button pressed?\n\nMultiD is waiting for trigger"
              n47 = event-data() -> ()  [unwired: 1 in, 6 out]
              n48 = Bundle("Enum"=CameraControlTypeDef."Trigger Source", "Value"=w507) -> (w508:cluster{"Enum":T8, "Value":T1})  [unwired: 1 in]
              n49 = Bundle("Mode"=w510, "Value"=w507) -> (w509:cluster{"Mode":T7, "Value":T1})  [unwired: 1 in]
              n50 = Enqueue Element(queue=w513, element=w508) -> ()  [unwired: 2 in, 3 out]
              n51 = Enqueue Element(queue=w512, element=w509) -> ()  [unwired: 2 in, 3 out]
            }
            event Value Change {
              n52 = event-data() -> ()  [unwired: 1 in, 6 out]
              n53 = Bundle("Enum"=CameraControlTypeDef."Readout Mode", "Value"=w515) -> (w514:cluster{"Enum":T8, "Value":T1})  [unwired: 1 in]
              n54 = Enqueue Element(queue=w517, element=w514) -> ()  [unwired: 2 in, 3 out]
            }
            event Value Change {
              w522 = ModeEnum."generateWaves"  # Mode
              n55 = event-data() -> ()  [unwired: 1 in, 6 out]
              n56 = Bundle("Mode"=w522, "Value"=w520) -> (w521:cluster{"Mode":T7, "Value":T1})  [unwired: 1 in]
              n57 = Enqueue Element(queue=w519, element=w521) -> ()  [unwired: 2 in, 3 out]
            }
            event Value Change {
              w528 = ModeEnum."generateWaves"  # Mode
              n58 = event-data() -> ()  [unwired: 1 in, 6 out]
              n59 = Bundle("Enum"=CameraControlTypeDef."Update", "Value"=w525) -> (w526:cluster{"Enum":T8, "Value":T1})  [unwired: 1 in]
              n60 = Bundle("Mode"=w528, "Value"=w525) -> (w527:cluster{"Mode":T7, "Value":T1})  [unwired: 1 in]
              n61 = Enqueue Element(queue=w524, element=w526) -> ()  [unwired: 2 in, 3 out]
              n62 = Enqueue Element(queue=w523, element=w527) -> ()  [unwired: 2 in, 3 out]
            }
            event "Signals Debugger": Value Change {
              n63 = event-data() -> ()  [unwired: 1 in, 6 out]
              n64 = disable-structure shown="Disabled" {
                frame Disabled {
                  n65 = control-ref of="stop"() -> (w533:refnum<vi>)
                  n66 = call "PopOutGraph.vi"("OK Button 2"=w533) -> ()  [unwired: 2 in]
                }
                frame Enabled {
                }
              }
              n67 = vi-ref "Graph.vi"() -> (w530:refnum<vi>)
              n68 = invoke class="VI" method="FP.Open"(reference=w530, "Activate"=TRUE ("Front Panel Window:Open"), "State"=T12."Standard") -> ()  [unwired: 2 in, 5 out]
            }
            event "Scan": Value Change {
              n69 = event-data() -> ("NewVal"=w534:bool)  [unwired: 1 in, 5 out]
              n70 = case shown="True" w534 {
                tunnel: w537 -> [_ w543]
                tunnel: [w538 w542] -> w536
                tunnel: w535 -> [w538 w541]
                frame False {
                }
                frame True {
                  w540 = ModeEnum."runWaves"  # Mode
                  n71 = Bundle("Mode"=w540, "Value"=w543) -> (w539:cluster{"Mode":T7, "Value":T1})  [unwired: 1 in]
                  n72 = Enqueue Element(queue=w541, element=w539) -> (queue out=w542:refnum<queue>)  [unwired: 2 in, 2 out]
                }
              }
            }
            event Timeout {
              n73 = event-data() -> ()  [unwired: 1 in, 3 out]
              n74 = property on="Microscope Settings" class="Clust (strict)"() -> ("Value"=w544:T1)  [unwired: 2 in, 2 out]
            }
          }
        }
        n75 = while "Camera Consumer" {
          tunnel: w154 -> [w326]
          tunnel: [w311] -> w158
          tunnel: w147 -> [w319]
          tunnel: [w327] -> w157
          shift-right: [w325] -> _
          shift-left: CameraControlTypeDef."Preview" ("Enum") -> [w315]
          tunnel: [w322] -> w152
          tunnel: w151 -> [w321]
          tunnel: w149 -> [w314]
          shift-right: [w323] -> w161
          shift-left: w162 -> [w324]
          stop <- w310 stop-if-true
          n76 = Dequeue Element(queue=w319, timeout in ms (-1)=1) -> (queue out=w318:refnum<queue>, element=w313:cluster{"Enum":T8, "Microscope Settings":T1}, timed out?=w317:bool)  [unwired: 1 in, 1 out]
          n77 = case shown="True" w317 {
            tunnel: [w329 CameraControlTypeDef."Preview" ("Enum")] -> w316
            tunnel: w315 -> [_ _]
            tunnel: w313 -> [w330 _]
            tunnel: [w328 _] -> w312
            frame False {
              n78 = Unbundle(w330) -> ("Enum"=w329:T8, "Microscope Settings"=w328:T1)
            }
            frame True {
            }
          }
          n79 = case shown="\"Readout Mode\"" w316 {
            selector: w316 -> [w335 w340 w345 w350 w355 w366 w371 w376 w381 w386 w414 w432 _ w461 _]
            tunnel: w318 -> [w334 w341 w346 w351 w356 w367 w372 w377 w382 w387 _ w428 w443 w463 w482]
            tunnel: [w334 w341 w346 w351 w356 w367 w372 w377 w382 w387 _ w428 w443 w463 w482] -> w327
            tunnel: w326 -> [w336 w339 w344 w349 w354 w365 w370 w375 w380 w385 w409 w431 w435 w460 w473]
            tunnel: [w336 w339 w344 w349 w354 w365 w370 w375 w380 w385 w395 w431 w434 w460 w474] -> w311
            tunnel: [w335 w340 w345 w350 w355 w366 w371 w376 w381 w386 w414 w432 CameraControlTypeDef."Preview" ("Enum") w461 w464] -> w325
            tunnel: w324 -> [w333 w338 w343 w348 w352 w363 w369 w374 w379 w384 w411 w430 w441 w462 w476]
            tunnel: [w333 w338 w343 w348 w352 w362 w369 w374 w379 w384 w388 w430 w439 w462 w475] -> w323
            tunnel: [w332 w337 w342 w347 w353 w364 w368 w373 w378 w383 w413 w429 w437 w459 w477] -> w322
            tunnel: w321 -> [w332 w337 w342 w347 w353 w364 w368 w373 w378 w383 w413 w429 w437 w459 _]
            tunnel: w314 -> [_ _ _ _ _ _ _ _ _ _ _ _ w436 _ _]
            tunnel: w312 -> [_ _ _ _ _ w361 _ _ _ _ w408 _ _ _ w466]
            frame "Idle" {
            }
            frame "IntervalLineInt" {
            }
            frame "Ram Record" {
            }
            frame "HardDisk Record" {
            }
            frame "Disengage Update" {
            }
            frame "Update", Default {
              w358 = u32 2049184 items=["SENSOR MODE"=4212128, "CCD MODE"=4212384, "READOUT MODE"=4211872, "ACTIVE VIEW INDEX"=4343136, "BITS PER CHANNEL"=4342976, "IMAGE PIXEL TYPE"=4343296, "BINNING"=4215968, "EXPOSURE TIME"=2049184, "CONTRAST GAIN"=3163312, "CONTRAST OFFSET"=3163328, "LIGHT MODE"=2114720, "SENSITIVITY"=2114992, "PHOTON IMAGING MODE"=2115200, "HIGH DYNAMIC RANGE MODE"=3163360, "WHITE BALANCE"=3163568, "TEMPERATURE"=2115232, "TEMPERATURE TARGET"=2115264, "SENSOR COOLER FAN"=2115296, "LINEBUNDLE HEIGHT"=4212192, "MECHANICAL SHUTTER"=2115488, "BACK FOCUS POSITION"=8422304, "TRIGGER CONNECTOR"=1066432, "TRIGGER SOURCE"=1066144, "OUTPUT TRIGGER SOURCE"=1852576, "TRIGGER GLOBAL EXPOSURE"=2049680, "FIRST TRIGGER BEHAVIOR"=2049696, "CHANNEL SYNC"=1852352, "READOUT DIRECTION"=4211904, "PRE HSYNC COUNT"=1852704, "INTERNAL LINE SPEED"=4226000, "INTERNAL LINE INTERVAL"=4226016] ("Parameter")
              n80 = Unbundle By Name(w361) -> ("Exposure/ms"=w360:dbl)  [unwired: 1 out]
              n81 = Divide(x=w360, y=1000.0) -> (x/y=w357:dbl)
              n82 = call "tm_setparameter_a.vi"("Value in"=w357, "Parameter"=w358, "Handle in"=w363) -> ("Handle out"=w362:u32)  [unwired: 7 in, 1 out]
            }
            frame "ROI" {
            }
            frame "Binning" {
            }
            frame "Scan Mode" {
            }
            frame "Trigger Mode" {
            }
            frame "Readout Mode" {
              w394 = u32 4194832  # Sensor Mode
              w398 = u32 2031888  # Exposure time
              n83 = Unbundle By Name(w408) -> ("Exposure/ms"=w407:dbl, "Slit.Slit Width /%"=w403:dbl, "Slit.Scanning Mode"=w392:dbl)
              n84 = call "tm_stopcapture.vi"("error in (no error)"=w409, "Handle in"=w411) -> ("error out"=w412:errorcluster, "Handle out"=w410:u32)  [unwired: 8 in]
              n85 = Divide(x=w407, y=1000.0) -> (x/y=w405:dbl)
              n86 = Multiply(x=w403, y=2048 ("input variable")) -> (x*y=w402:dbl)
              n87 = call "tm_unpreparecapture.vi"("error in (no error)"=w412, "Handle in"=w410) -> ("error out"=w389:errorcluster, "Handle out"=w393:u32)  [unwired: 8 in]
              n88 = call "tm_setpropertyvalue.vi"("error in (no error)"=w389, "Value in"=w392, "Property ID"=w394, "Handle in"=w393) -> ("error out"=w390:errorcluster, "Handle out"=w391:u32)  [unwired: 6 in]
              n89 = Divide(x=w402, y=100.0) -> (x/y=w400:dbl)
              n90 = case shown="12" w392 {
                tunnel: [w417 w418] -> w399
                tunnel: w405 -> [w417 w426]
                tunnel: w400 -> [_ w425]
                tunnel: w391 -> [w416 w420]
                tunnel: [w416 w422] -> w397
                tunnel: [w415 w421] -> w396
                tunnel: w390 -> [w415 w419]
                frame 1, Default {
                }
                frame 12 {
                  w424 = u32 4208720  # Line Interval
                  n91 = formula code="slitExpos=frameInter*LW/(LinesToReadout\n+10+LW);\nlineInter = slitExpos / LW;"("frameInter"=w426, "LW"=w425, "LinesToReadout"=2048 ("input variable")) -> ("slitExpos"=w418:dbl, "lineInter"=w423:dbl)
                  n92 = call "tm_setpropertyvalue.vi"("error in (no error)"=w419, "Value in"=w423, "Property ID"=w424, "Handle in"=w420) -> ("error out"=w421:errorcluster, "Handle out"=w422:u32)  [unwired: 6 in]
                }
              }
              n93 = call "tm_setpropertyvalue.vi"("error in (no error)"=w396, "Value in"=w399, "Property ID"=w398, "Handle in"=w397) -> ("error out"=w395:errorcluster, "Handle out"=w388:u32)  [unwired: 6 in]
            }
            frame "Readout Direction" {
            }
            frame "Preview" {
              n94 = call "tm_waitnextframe.vi"("error in (no error)"=w435, "Timeout"=500, "Handle in"=w441) -> ("error out"=w433:errorcluster, "Handle out"=w440:u32)  [unwired: 5 in, 2 out]
              n95 = case shown="No Error" w433 {
                selector: w433 -> [w444 w458]
                tunnel: w440 -> [w456 w457]
                tunnel: [w455 w457] -> w439
                tunnel: w437 -> [w454 _]
                tunnel: w436 -> [w453 _]
                tunnel: w435 -> [w448 _]
                tunnel: [w445 w458] -> w434
                frame No Error {
                  w450 = 0 ("Timeout")
                  n96 = call "tm_getframe_a.vi"("error in (no error)"=w444, "Buffer Info"=w454, "Handle in"=w456) -> ("error out"=w446:errorcluster, "Data 16"=w451:u16[][], "Handle out"=w455:u32)  [unwired: 4 in, 2 out]
                  n97 = Bundle("State"=Stack_Track."Display", "Timeout"=w450, "Data 16"=w451, "Timeout"=w450) -> (w449:T14)  [unwired: 1 in]
                  n98 = Enqueue Element(queue=w453, element=w449, error in (no error)=w448) -> (error out=w447:errorcluster)  [unwired: 1 in, 2 out]
                  n99 = Merge Errors(w446, w447) -> (w445:errorcluster)
                }
                frame Error {
                }
              }
            }
            frame "ROIWindow" {
            }
            frame "Trigger Source" {
              (unwired) u32 1066144 items=["SENSOR MODE"=4212128, "CCD MODE"=4212384, "READOUT MODE"=4211872, "ACTIVE VIEW INDEX"=4343136, "BITS PER CHANNEL"=4342976, "IMAGE PIXEL TYPE"=4343296, "BINNING"=4215968, "EXPOSURE TIME"=2049184, "CONTRAST GAIN"=3163312, "CONTRAST OFFSET"=3163328, "LIGHT MODE"=2114720, "SENSITIVITY"=2114992, "PHOTON IMAGING MODE"=2115200, "HIGH DYNAMIC RANGE MODE"=3163360, "WHITE BALANCE"=3163568, "TEMPERATURE"=2115232, "TEMPERATURE TARGET"=2115264, "SENSOR COOLER FAN"=2115296, "LINEBUNDLE HEIGHT"=4212192, "MECHANICAL SHUTTER"=2115488, "BACK FOCUS POSITION"=8422304, "TRIGGER CONNECTOR"=1066432, "TRIGGER SOURCE"=1066144, "OUTPUT TRIGGER SOURCE"=1852576, "TRIGGER GLOBAL EXPOSURE"=2049680, "FIRST TRIGGER BEHAVIOR"=2049696, "CHANNEL SYNC"=1852352, "READOUT DIRECTION"=4211904, "PRE HSYNC COUNT"=1852704, "INTERNAL LINE SPEED"=4226000, "INTERNAL LINE INTERVAL"=4226016] ("Parameter")
              w472 = 1 items=["Snap", "Sequence"] ("Capture mode")
              n100 = Unbundle By Name(w466) -> ("Mode"=w465:enum16{"X", "XY", "XYZ", "XYZT", "XYZC"})
              n101 = call "tm_stopcapture.vi"("error in (no error)"=w473, "Handle in"=w476) -> ("error out"=w480:errorcluster, "Handle out"=w481:u32)  [unwired: 8 in]
              n102 = call "tm_unpreparecapture.vi"("error in (no error)"=w480, "Handle in"=w481) -> ("error out"=w468:errorcluster, "Handle out"=w471:u32)  [unwired: 8 in]
              n103 = case shown="\"XYZT\"" w465 {
                tunnel: [T9 {"Mode"=2, "Polarity"=2, "Times"=2, "Delay"=0.0} ("Parameters") T9 {"Mode"=2, "Polarity"=2, "Times"=2, "Delay"=0.0} ("Parameters") T9 {"Mode"=2, "Polarity"=2, "Times"=2, "Delay"=0.0} ("Parameters") T9 {"Mode"=1, "Polarity"=2, "Times"=2, "Delay"=0.0} ("Parameters") T9 {"Mode"=1, "Polarity"=2, "Times"=2, "Delay"=0.0} ("Parameters")] -> w469
                tunnel: [CameraControlTypeDef."Preview" ("Enum") CameraControlTypeDef."Idle" ("Enum") CameraControlTypeDef."Idle" ("Enum") CameraControlTypeDef."Idle" ("Enum") CameraControlTypeDef."Preview" ("Enum")] -> w464
                frame "XY", Default {
                }
                frame "XYZT" {
                }
                frame "XYZ" {
                }
                frame "XYZC" {
                }
                frame "X" {
                }
              }
              n104 = call <userlib>:"tm_setinputtrigger.vi"("error in (no error)"=w468, "Parameters"=w469, "Handle in"=w471) -> ("error out"=w467:errorcluster, "Handle out"=w470:u32)  [unwired: 7 in]
              n105 = call "tm_preparecapture.vi"("error in (no error)"=w467, "Capture mode"=w472, "Handle in"=w470) -> ("error out"=w479:errorcluster, "Buffer Info"=w477:T5, "Handle out"=w478:u32)  [unwired: 5 in, 1 out]
              n106 = call "tm_startcapture_b.vi"("error in (no error)"=w479, "Handle in"=w478) -> ("error out"=w474:errorcluster, "Handle out"=w475:u32)  [unwired: 8 in]
            }
          }
          n107 = local read "stop"() -> (w310:bool)
        }
        n108 = while {
          tunnel: w139 -> [w180]
          shift-right: [w176] -> _
          shift-left: _ -> [w175]
          tunnel: w146 -> [w174]
          shift-right: [w170] -> w140
          shift-left: w143 -> [w169]
          shift-right: [w173] -> _
          shift-left: w145 -> [w172]
          shift-right: [w168] -> w141
          shift-left: w142 -> [w167]
          tunnel: [w166] -> w138
          shift-right: [w165] -> w137
          shift-left: _ -> [w164]
          stop <- w163 stop-if-true
          n109 = Dequeue Element(queue=w180, timeout in ms (-1)=1) -> (queue out=w166:refnum<queue>, element=w179:cluster{"Mode":T7, "Microscope Settings":T1})  [unwired: 1 in, 2 out]
          n110 = Unbundle(w179) -> ("Mode"=w178:T7, "Microscope Settings"=w177:T1)
          n111 = case shown="\"Idle\", Default" w178 {
            tunnel: [_ _ _ TRUE] -> _
            tunnel: w177 -> [_ w197 w263 _]
            tunnel: [w185 w198 w262 w284] -> w176
            tunnel: w175 -> [w185 w189 w262 w284]
            tunnel: w174 -> [_ _ _ _]
            tunnel: w166 -> [_ w188 w264 _]
            tunnel: [w182 w193 w242 w283] -> w168
            tunnel: [w183 w191 w257 w282] -> w170
            tunnel: w169 -> [w183 w190 w265 w282]
            tunnel: [w184 w196 w244 w281] -> w173
            tunnel: w172 -> [w184 w195 w244 w281]
            tunnel: w167 -> [w182 w194 w253 w283]
            tunnel: [w181 w187 w239 w279] -> w165
            tunnel: w164 -> [w181 w187 w238 w279]
            frame "Idle", Default {
            }
            frame "generateWaves" {
              n112 = Unbundle By Name(w197) -> ("Mode"=w192:enum16{"X", "XY", "XYZ", "XYZT", "XYZC"})
              n113 = case shown="\"XY\", Default" w192 {
                tunnel: [w203 w224] -> w198
                tunnel: w197 -> [_ w209]
                tunnel: [w201 w215] -> w196
                tunnel: w195 -> [w201 _]
                tunnel: w194 -> [w202 w230]
                tunnel: [w202 w230] -> w193
                tunnel: [w199 w229] -> w191
                tunnel: w190 -> [w200 w229]
                tunnel: w189 -> [w203 _]
                tunnel: w188 -> [_ _]
                tunnel: [_ w210] -> w186
                frame "X" {
                  n114 = call "Calibration.vi"("Analogue In"=w200) -> ("Analogue In Out"=w199:refnum<k21>)
                }
                frame "XY", Default {
                  w212 = 10.0  # Piezo Factor
                  # "XY Mirrors"
                  n115 = Unbundle By Name(w209) -> ("Piezo Position /um"=w204:dbl, "Exposure/ms"=w206:dbl, "Samples per millisecond"=w205:dbl, "Camera Delay"=w207:dbl, "Relax/ms"=w208:dbl)
                  n116 = Unbundle By Name(w209) -> ()  [unwired: 1 out]
                  n117 = Divide(x=w204, y=w212) -> (x/y=w211:dbl)
                  n118 = call "XY Galvo With Homography.vi"("Exposure (ms)"=w206, "Camera Delay /ms"=w207, "Samples /Millisecond"=w205, "Relax (ms)"=w208, "Piezo Position (um)"=w211) -> ("Scan Mirror Signal"=w234:dbl[], "Piezo Signal"=w228:dbl[], "Camera Signal"=w217:dbl[], "Laser Signal"=w222:dbl[], "Z Mirror Signal"=w233:dbl[])  [unwired: 10 in]
                  n119 = Divide(x=0.001 ("y"), y=w205) -> (x/y=w216:dbl)
                  n120 = Bundle By Name("Y"=w234, "dt"=w216) -> (w231:waveform(dbl))  [unwired: 1 in]
                  n121 = Bundle By Name("Y"=w228, "dt"=w216) -> (w227:waveform(dbl))  [unwired: 1 in]
                  n122 = Bundle By Name("Y"=w233, "dt"=w216) -> (w232:waveform(dbl))  [unwired: 1 in]
                  n123 = Build Array(w217) -> (w218:dbl[][])
                  n124 = Build Array(w222) -> (w225:dbl[][])
                  n125 = Transpose 2D Array(2D array=w218) -> (transposed array=w220:dbl[][])
                  n126 = Transpose 2D Array(2D array=w225) -> (transposed array=w221:dbl[][])
                  n127 = Bundle By Name("data"=w220) -> (w219:digitaldata)  [unwired: 1 in]
                  n128 = Bundle By Name("data"=w221) -> (w223:digitaldata)  [unwired: 1 in]
                  n129 = Bundle By Name("Y"=w219, "dt"=w216) -> (w214:digitalwaveform)  [unwired: 1 in]
                  n130 = Bundle By Name("Y"=w223, "dt"=w216) -> (w213:digitalwaveform)  [unwired: 1 in]
                  n131 = Build Array(w231, w232, w227) -> (w224:waveform(dbl)[])
                  n132 = Build Array(w214, w213) -> (w215:digitalwaveform[])
                  n133 = Bundle(w224, "Digital Waveform"=w214, "Digital Waveform"=w213) -> (w210:T15)  [unwired: 1 in]
                }
              }
              n134 = call "Graph.vi"("Cluster"=w186) -> ()
            }
            frame "runWaves" {
              n135 = Unbundle By Name(w263) -> ("Samples per millisecond"=w235:dbl)
              n136 = Index Array(array=w262, index=0) -> (element=w260:waveform(dbl))
              n137 = Multiply(x=w235, y=1000.0) -> (x*y=w255:dbl)
              n138 = local read "Scan Continuously"() -> (w256:bool)
              n139 = call-poly <vilib>:"Number of Waveform Samples.vi"("waveform in"=w260) -> ("number of samples"=w236:i32)  [unwired: 8 in, 2 out]
              n140 = call-poly <vilib>:"DAQmx Timing.vi"("task/channels in"=w265, "samples per channel"=w236, "rate"=w255, "error in"=w238) -> ("task out"=w268:refnum<k21>, "error out"=w259:errorcluster)  [unwired: 10 in]
              n141 = call-poly <vilib>:"DAQmx Timing.vi"("task/channels in"=w253, "samples per channel"=w236, "rate"=w255, "error in"=w238) -> ("task out"=w254:refnum<k21>, "error out"=w251:errorcluster)  [unwired: 10 in]
              n142 = case shown="True" w256 {
                tunnel: w264 -> [w270 w278]
                tunnel: [w271 w277] -> _
                tunnel: w263 -> [w272 w276]
                frame False {
                  n143 = Bundle("Mode"=ModeEnum."Idle", "Microscope Settings"=w272) -> (w273:cluster{"Mode":T7, "Microscope Settings":T1})  [unwired: 1 in]
                  n144 = Enqueue Element(queue=w270, element=w273) -> (queue out=w271:refnum<queue>)  [unwired: 2 in, 2 out]
                }
                frame True {
                  n145 = Bundle("Mode"=ModeEnum."runWaves", "Microscope Settings"=w276) -> (w275:cluster{"Mode":T7, "Microscope Settings":T1})  [unwired: 1 in]
                  n146 = Enqueue Element(queue=w278, element=w275) -> (queue out=w277:refnum<queue>)  [unwired: 2 in, 2 out]
                }
              }
              n147 = call-poly <vilib>:"DAQmx Write.vi"("task/channels in"=w268, "data"=w262, "error in"=w259) -> ("task out"=w246:refnum<k21>, "error out"=w249:errorcluster)  [unwired: 10 in, 1 out]
              n148 = call-poly <vilib>:"DAQmx Write.vi"("task/channels in"=w254, "data"=w244, "error in"=w251) -> ("task out"=w245:refnum<k21>, "error out"=w248:errorcluster)  [unwired: 10 in, 1 out]
              n149 = Merge Errors(w249, w248) -> (w247:errorcluster)
              n150 = call <vilib>:"DAQmx Start Task.vi"("task/channels in"=w246, "error in"=w247) -> ("task out"=w267:refnum<k21>, "error out"=w266:errorcluster)  [unwired: 12 in]
              n151 = call <vilib>:"DAQmx Start Task.vi"("task/channels in"=w245, "error in"=w247) -> ("task out"=w252:refnum<k21>, "error out"=w250:errorcluster)  [unwired: 12 in]
              n152 = call <vilib>:"DAQmx Wait Until Done.vi"("task/channels in"=w267, "error in"=w266) -> ("task out"=w258:refnum<k21>, "error out"=w241:errorcluster)  [unwired: 12 in]
              n153 = call <vilib>:"DAQmx Wait Until Done.vi"("task/channels in"=w252, "error in"=w250) -> ("task out"=w243:refnum<k21>, "error out"=w240:errorcluster)  [unwired: 12 in]
              n154 = call <vilib>:"DAQmx Stop Task.vi"("task/channels in"=w258) -> ("task out"=w257:refnum<k21>)  [unwired: 13 in, 1 out]
              n155 = Merge Errors(w241, w240) -> (w239:errorcluster)
              n156 = call <vilib>:"DAQmx Stop Task.vi"("task/channels in"=w243) -> ("task out"=w242:refnum<k21>)  [unwired: 13 in, 1 out]
            }
            frame "stop" {
            }
          }
          n157 = local read "stop"() -> (w163:bool)
        }
        n158 = while "Tiff Consumer" {
          tunnel: [w288] -> w159
          tunnel: [w291] -> w156
          tunnel: w149 -> [w293]
          tunnel: w148 -> [w285]
          stop <- w295 stop-if-true
          # "Delay, maybe?\nCheck"
          n159 = Dequeue Element(queue=w293, timeout in ms (-1)=1) -> (queue out=w290:refnum<queue>, element=w292:T10, error out=w289:errorcluster)  [unwired: 1 in, 1 out]
          n160 = Unbundle By Name(w292) -> ("State"=w286:T11, "Image"=w287:u16[][])  [unwired: 1 out]
          n161 = case shown="\"Idle\", Default" w286 {
            selector: w286 -> [_ w306 w307]
            tunnel: [w303 w305 w308] -> w291
            tunnel: w290 -> [w303 w305 w308]
            tunnel: [Stack_Track."Idle" ("State") w306 w307] -> _
            tunnel: w287 -> [w298 _ _]
            tunnel: w285 -> [w302 _ _]
            tunnel: w289 -> [w301 w304 w309]
            tunnel: [w300 w304 w309] -> w288
            frame "Display" {
              n162 = call "IMAQ ArrayToImage"("Image Pixels (U16)"=w298, "error in (no error)"=w301, "Image"=w302) -> ("error out"=w300:errorcluster, "Image Out"=w297:T3)  [unwired: 7 in]
              "Image" <- w297
              n163 = call "IMAQ Histograph"("Image"=w297) -> ("Histogram Graph"=→"Histogram":T4)  [unwired: 7 in, 3 out]
            }
            frame "Idle", Default {
            }
            frame "Start Sequence" {
            }
          }
          n164 = local read "stop"() -> (w295:bool)
        }
        n165 = Merge Errors(w158, w159, w137) -> (w160:errorcluster)
      }
      frame "deinit" {
        n166 = call <vilib>:"DAQmx Stop Task.vi"("task/channels in"=w555) -> ("task out"=w556:refnum<k21>)  [unwired: 13 in, 1 out]
        n167 = call <vilib>:"DAQmx Stop Task.vi"("task/channels in"=w557) -> ("task out"=w558:refnum<k21>)  [unwired: 13 in, 1 out]
        n168 = call <vilib>:"DAQmx Clear Task.vi"("task in"=w556) -> ("error out"=w552:errorcluster)  [unwired: 14 in]
        n169 = call "tm_stopcapture.vi"("error in (no error)"=w567, "Handle in"=w563) -> ("error out"=w570:errorcluster, "Handle out"=w569:u32)  [unwired: 8 in]
        n170 = call <vilib>:"DAQmx Clear Task.vi"("task in"=w558) -> ("error out"=w553:errorcluster)  [unwired: 14 in]
        n171 = call "tm_unpreparecapture.vi"("error in (no error)"=w570, "Handle in"=w569) -> ("error out"=w571:errorcluster, "Handle out"=w568:u32)  [unwired: 8 in]
        n172 = call "tm_closecamera.vi"("error in (no error)"=w571, "Handle in"=w568) -> ("error out"=w572:errorcluster)  [unwired: 9 in]
        n173 = Flush Queue(queue=w545) -> (queue out=w551:refnum<queue>)  [unwired: 1 in, 2 out]
        n174 = call "tm_deinitialize.vi"("error in (no error)"=w572) -> ("error out"=w548:errorcluster)  [unwired: 10 in]
        n175 = Release Queue(queue=w546, error in (no error)=w548) -> (error out=w565:errorcluster)  [unwired: 1 in, 2 out]
        n176 = Release Queue(queue=w551) -> (error out=w554:errorcluster)  [unwired: 2 in, 2 out]
        n177 = Flush Queue(queue=w550, error in (no error)=w548) -> (queue out=w549:refnum<queue>, error out=w547:errorcluster)  [unwired: 1 out]
        n178 = Release Queue(queue=w549, error in (no error)=w547) -> (error out=w564:errorcluster)  [unwired: 1 in, 2 out]
        n179 = Merge Errors(w565, w564, w554, w553, w552) -> (w566:errorcluster)
      }
    }
    n180 = Or(x="stop", y=w17) -> (x .or. y?=w18:bool)
  }
  "error IO" <- w5
  n181 = disable-structure shown="Enabled" {
    frame Disabled {
      # "Parallise decode buffer"
      n182 = call "tm_startcapture_b.vi"() -> ()  [unwired: 10 in, 2 out]
      n183 = call "tm_waitnextframe.vi"() -> ()  [unwired: 8 in, 4 out]
      n184 = call "tm_getframe_a.vi"() -> ()  [unwired: 7 in, 5 out]
    }
    frame Enabled {
    }
  }
